vi "Render Children.vi"(8 "Error In":errorcluster, 10 "Children":refnum<class "Node.lvclass">[](array[class]), 11 "Renderer In":refnum<class "Renderer.lvclass">) -> (0 "Error Out":errorcluster, 2 "Output":string, 3 "Renderer Out":refnum<class "Renderer.lvclass">)   [LabVIEW 2018, in "Toolkit.lvlib" / "Renderer.lvclass"]
uses:
  Renderer.lvclass
  Nodes/Node/Node.lvclass
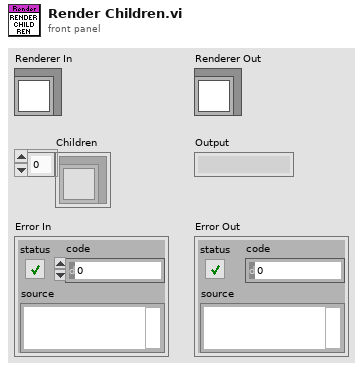
[diagram p1: front panel]
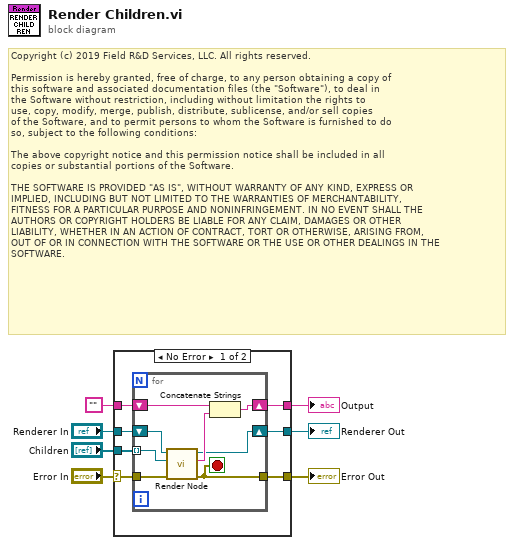
[diagram p0: block diagram]
diagram:
  # "Copyright (c) 2019 Field R&D Services, LLC. All rights reserved.\n\nPermission is hereby granted, free of charge, to any person obtaining a copy of\nthis software and associated documentation files (the \"Software\"), to deal in\nthe Software without restriction, including without limitation the rights to\nuse, copy, modify, merge, publish, distribute, sublicense, and/or sell copies\nof the Software, and to permit persons to whom the Software is furnished to do\nso, subject to the following conditions:\n\nThe above copyright notice and this permission notice shall be included in all\ncopies or substantial portions of the Software.\n\nTHE SOFTWARE IS PROVIDED \"AS IS\", WITHOUT WARRANTY OF ANY KIND, EXPRESS OR\nIMPLIED, INCLUDING BUT NOT LIMITED TO THE WARRANTIES OF MERCHANTABILITY,\nFITNESS FOR A PARTICULAR PURPOSE AND NONINFRINGEMENT. IN NO EVENT SHALL THE\nAUTHORS OR COPYRIGHT HOLDERS BE LIABLE FOR ANY CLAIM, DAMAGES OR OTHER\nLIABILITY, WHETHER IN AN ACTION OF CONTRACT, TORT OR OTHERWISE, ARISING FROM,\nOUT OF OR IN CONNECTION WITH THE SOFTWARE OR THE USE OR OTHER DEALINGS IN THE\nSOFTWARE."
  n1 = case shown="No Error" "Error In" {
    selector: "Error In" -> [w9 w23]
    tunnel: [w14 w25] -> w7
    tunnel: [w13 w23] -> w6
    tunnel: [w12 w24] -> w1
    tunnel: "Renderer In" -> [w8 w24]
    tunnel: "Children" -> [w11 _]
    tunnel: "" -> [w10 w25]
    frame No Error {
      n2 = for {
        tunnel: w9 -> [w15]
        tunnel: w11 -> [w20] mode=indexing
        tunnel: [w16] -> w13
        shift-right: [w21] -> w14
        shift-left: w10 -> [w22]
        shift-right: [w17] -> w12
        shift-left: w8 -> [w19]
        stop <- w16 stop-if-true
        n3 = call "Render Node.vi"("Error In"=w15, "Node"=w20, "Renderer In"=w19) -> ("Error Out"=w16:errorcluster, "Output"=w18:string, "Renderer Out"=w17:refnum<class "Renderer.lvclass">)  [unwired: 6 in]
        n4 = Concatenate Strings(w22, w18) -> (w21:string)
      }
    }
    frame Error {
    }
  }
  "Output" <- w7
  "Error Out" <- w6
  "Renderer Out" <- w1
